vi "Status.vi"(0 "VISA Refnum in":refnum<visa-resource-name>, 11 "Error In":errorcluster) -> (4 "VISA Refnum out":refnum<visa-resource-name>, 6 "Voltage":string, 15 "Error Out":errorcluster)   [LabVIEW 2025]
panel:
  out "read buffer":string
  out "return count":u32
  out "Command":string
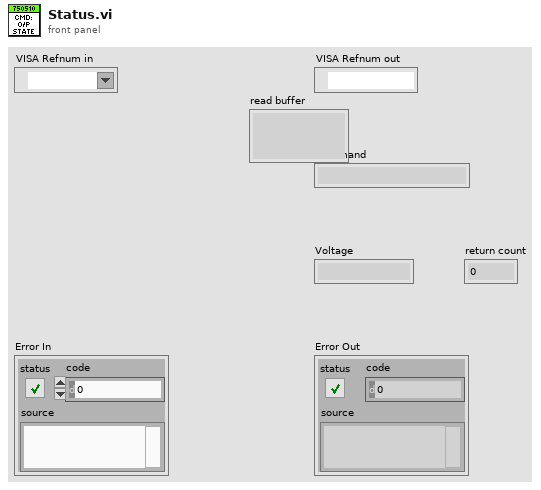
[diagram p1: front panel]
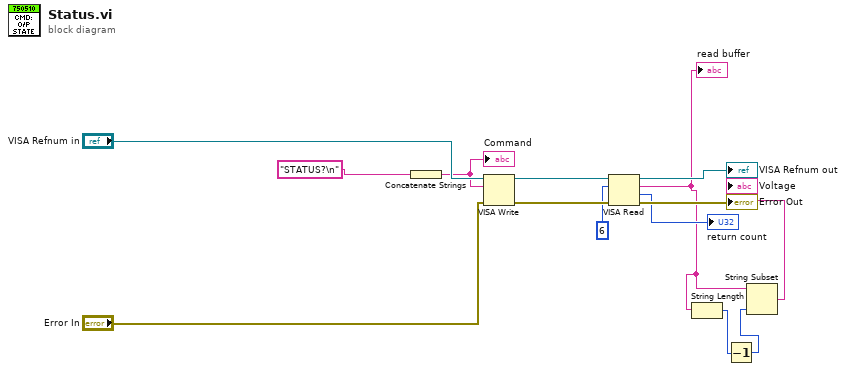
[diagram p0: block diagram]
diagram:
  n1 = Concatenate Strings("STATUS?\n") -> (w8:string)
  "Command" <- w8
  n2 = VISA Write(VISA resource name="VISA Refnum in", write buffer=w8, error in (no error)="Error In") -> (VISA resource name out=w10:refnum<visa-resource-name>, error out=w11:errorcluster)  [unwired: 1 out]
  n3 = VISA Read(VISA resource name=w10, byte count=u32 6, error in (no error)=w11) -> (VISA resource name out=→"VISA Refnum out":refnum<visa-resource-name>, read buffer=w1:string, return count=→"return count":u32, error out=→"Error Out":errorcluster)
  "read buffer" <- w1
  n4 = String Length(string=w1) -> (length=w4:i32)
  n5 = Decrement(x=w4) -> (x-1=w3:i32)
  n6 = String Subset(string=w1, length (rest)=w3) -> (substring=→"Voltage":string)  [unwired: 1 in]
